vi "EOD Read1.vi"(8 "error in (no error)":errorcluster, 10 "size (in bytes)":i64, 11 "Byte Stream File in":refnum<file>) -> (0 "error out":errorcluster, 1 "EODDataOut":T1(array[cluster]), 2 "Iteration Number":i32, 3 "Byte Stream File out":refnum<file>)   [LabVIEW 2014]
panel:
  out "Wave Offset":i32[](array[numeric])
  # "EOD File Reader VI"
  # "Inputs"
  # "Outputs"
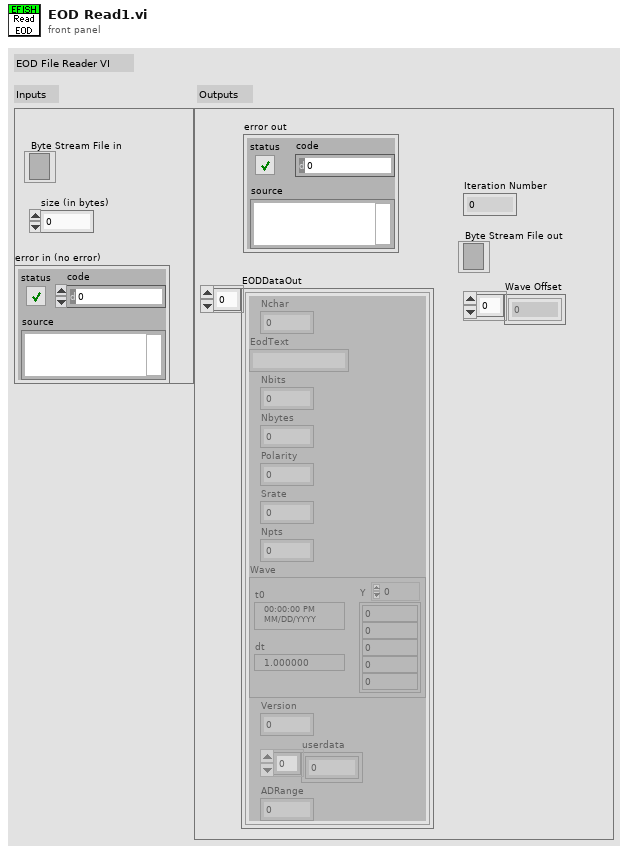
[diagram p1: front panel]
types:
  T1 = cluster{"Nchar":i32, "EodText":string, "Nbits":i32, "Nbytes":i32, "Polarity":i32, "Srate":i32, "Npts":i32, "Wave":waveform(dbl), "Version":i32, "userdata":dbl[], "ADRange":dbl}[]
  T2 = cluster{"Nchar":i32, "EodText":string, "Nbits":i32, "Nbytes":i32, "Polarity":i32, "Srate":i32, "Npts":i32, "Wave":waveform(dbl), "Version":i32, "userdata":dbl[], "ADRange":dbl}
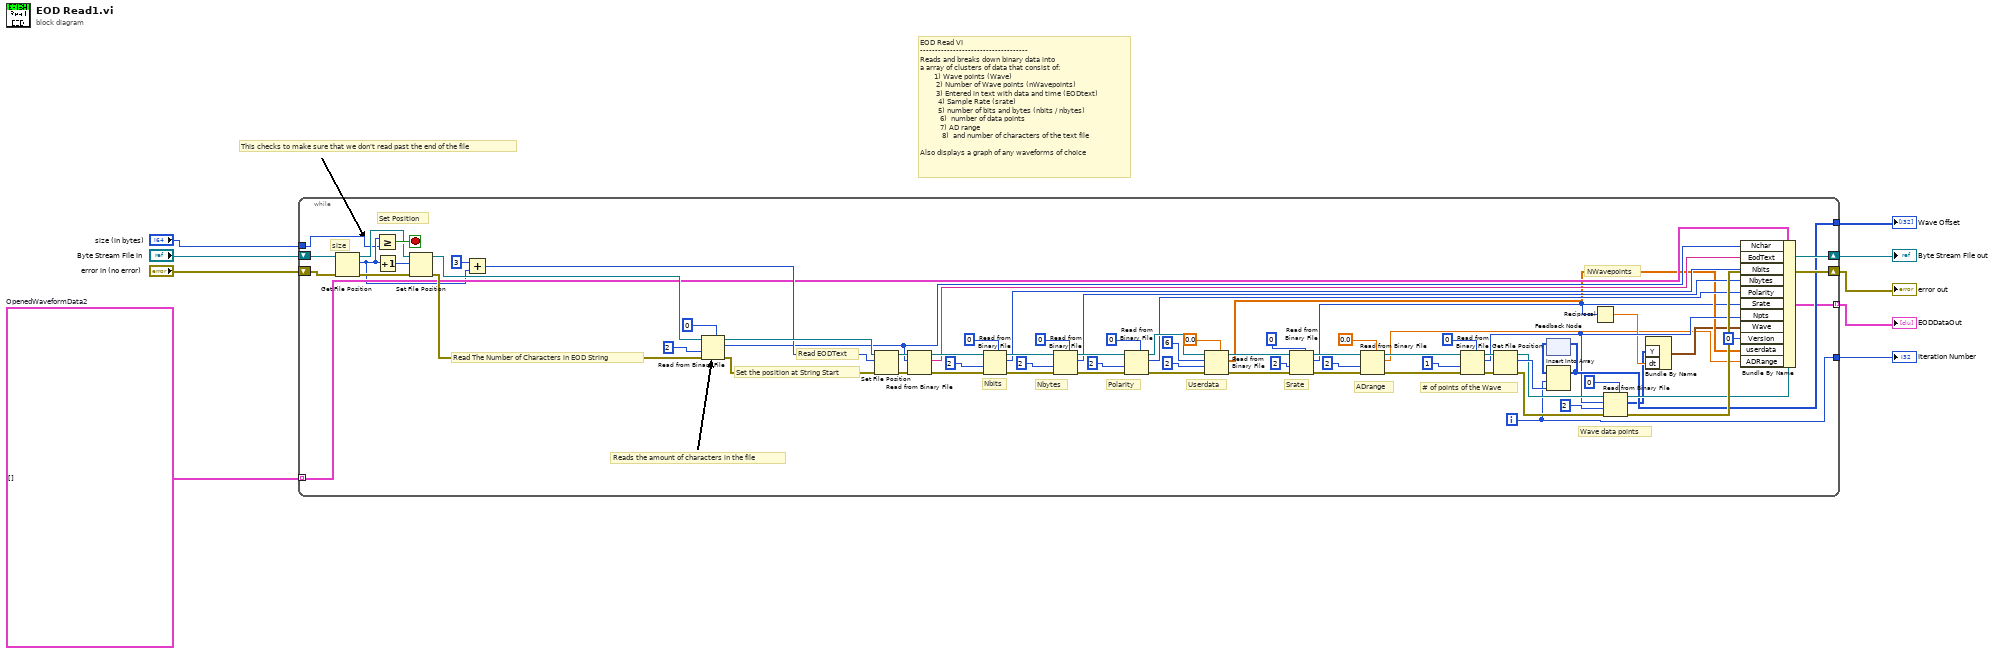
[diagram p0: block diagram]
diagram:
  w3 = T1 []  # OpenedWaveformData2
  # "This checks to make sure that we don't read past the end of the file"
  # "EOD Read VI\n------------------------------------\nReads and breaks down binary data into\na array of clusters of data that consist of:\n       1) Wave points (Wave)\n        2) Number of Wave points (nWavepoints)\n        3) Entered in text with data and time (EODtext)\n         4) Sample Rate (srate) \n         5) number of bits and bytes (nbits / nbytes)\n          6)  number of data points\n          7) AD range\n           8)  and number of characters of the text file\n\nAlso displays a graph of any waveforms of choice"
  n1 = while {
    shift-right: [w35] -> w7
    shift-left: "Byte Stream File in" -> [w43]
    shift-right: [w39] -> w8
    shift-left: "error in (no error)" -> [w40]
    tunnel: "size (in bytes)" -> [w10]
    tunnel: [w28] -> w6
    tunnel: [w27] -> w4
    tunnel: w3 -> [w26] mode=indexing
    tunnel: [w13] -> w2 mode=indexing
    i -> [w28]
    stop <- w44 stop-if-true
    # "ADrange"
    # "Nbits"
    # "Reads the amount of characters in the file"
    # "size"
    # "# of points of the Wave"
    # "Wave data points"
    # "NWavepoints"
    # "Srate"
    # "Userdata"
    # "Polarity"
    # "Nbytes"
    # "Read EODText"
    # "Set the position at String Start"
    # "Read The Number of Characters in EOD String"
    # "Set Position"
    n2 = Get File Position(4:w40, 7:w43) -> (0:w41:errorcluster, 2:w11:i64, 3:w42:refnum<file>)
    n3 = Greater Or Equal?(x=w11, y=w10) -> (x >= y?=w44:bool)
    n4 = Increment(x=w11) -> (x+1=w36:i64)
    n5 = Set File Position(offset (in bytes) (0)=w36, refnum=w42, error in=w41) -> (refnum out=w82:refnum<file>, error out=w54:errorcluster)  [unwired: 1 in]
    n6 = Add(x=3, y=w11) -> (x+y=w38:i64)
    n7 = Read from Binary File(5:u8 0, 8:w54, 9:2, 11:w82) -> (0:w53:errorcluster, 2:w23:u8, 3:w81:refnum<file>)  [unwired: 2 in, 1 out]
    n8 = Set File Position(offset (in bytes) (0)=w38, refnum=w81, error in=w53) -> (refnum out=w80:refnum<file>, error out=w52:errorcluster)  [unwired: 1 in]
    n9 = Read from Binary File(8:w52, 10:w23, 11:w80) -> (0:w51:errorcluster, 2:w24:string, 3:w79:refnum<file>)  [unwired: 3 in, 1 out]
    n10 = Read from Binary File(5:i8 0, 8:w51, 9:2, 11:w79) -> (0:w50:errorcluster, 2:w22:i8, 3:w56:refnum<file>)  [unwired: 2 in, 1 out]
    n11 = Read from Binary File(5:i8 0, 8:w50, 9:2, 11:w56) -> (0:w49:errorcluster, 2:w21:i8, 3:w57:refnum<file>)  [unwired: 2 in, 1 out]
    n12 = Read from Binary File(5:i8 0, 8:w49, 9:2, 11:w57) -> (0:w48:errorcluster, 2:w20:i8, 3:w55:refnum<file>)  [unwired: 2 in, 1 out]
    n13 = Read from Binary File(5:sgl 0.0, 8:w48, 9:2, 10:6, 11:w55) -> (0:w47:errorcluster, 2:w19:sgl[], 3:w76:refnum<file>)  [unwired: 1 in, 1 out]
    n14 = Read from Binary File(5:u32 0, 8:w47, 9:2, 11:w76) -> (0:w46:errorcluster, 2:w18:u32, 3:w68:refnum<file>)  [unwired: 2 in, 1 out]
    n15 = Read from Binary File(5:sgl 0.0, 8:w46, 9:2, 11:w68) -> (0:w45:errorcluster, 2:w14:sgl, 3:w63:refnum<file>)  [unwired: 2 in, 1 out]
    n16 = Read from Binary File(5:u32 0, 8:w45, 9:1, 11:w63) -> (0:w30:errorcluster, 2:w25:u32, 3:w32:refnum<file>)  [unwired: 2 in, 1 out]
    n17 = Get File Position(4:w30, 7:w32) -> (0:w29:errorcluster, 2:w34:i64, 3:w31:refnum<file>)
    n18 = feedback #1() -> (w33:i64[])  [unwired: 1 in]
    n19 = Insert Into Array(array=w33, index=w28, new element=w34) -> (w27:i64[])
    n20 = feedback-in #1(w27) -> ()
    n21 = Reciprocal(x=w18) -> (1/x=w17:dbl)
    n22 = Read from Binary File(5:i16 0, 8:w29, 9:2, 10:w25, 11:w31) -> (0:w39:errorcluster, 2:w16:i16[], 3:w35:refnum<file>)  [unwired: 1 in, 1 out]
    n23 = Bundle By Name("Y"=w16, "dt"=w17) -> (w15:waveform(i16))  [unwired: 1 in]
    n24 = Bundle By Name(cluster=w26, "Nchar"=w23, "EodText"=w24, "Nbits"=w22, "Nbytes"=w21, "Polarity"=w20, "Srate"=w18, "Npts"=w25, "Wave"=w15, "Version"=0, "userdata"=w19, "ADRange"=w14) -> (w13:T2)
  }
  "error out" <- w8
  "Byte Stream File out" <- w7
  "Iteration Number" <- w6
  "Wave Offset" <- w4
  "EODDataOut" <- w2
